vi "Close.vi"(8 "error in (no error)":errorcluster, 11 "Task Base in":refnum<class "Task Base.lvclass">) -> (0 "error out":errorcluster, 3 "Task Base out":refnum<class "Task Base.lvclass">)   [LabVIEW 2023, in "HAL GOOP4.lvlib" / "Task Base.lvclass"]
uses:
  Task Base.lvclass
  Task Base.lvclass/Task Base.ctl
  Measure and Stimulus Subsystems/Measure and Stimulus Subsystems.lvclass
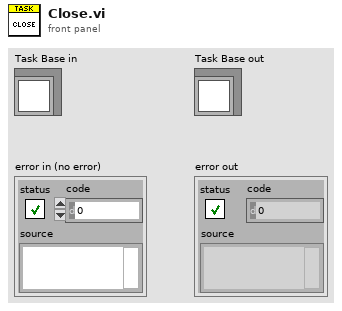
[diagram p1: front panel]
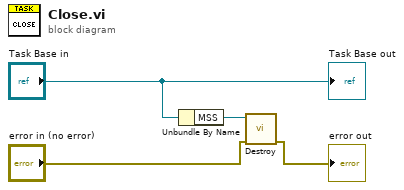
[diagram p0: block diagram]
diagram:
  n1 = Unbundle By Name("Task Base in") -> ("MSS"=w3:refnum<class "Measure and Stimulus Subsystems.lvclass">)
  n2 = call "Destroy.vi"("Error In"="error in (no error)", "reference in"=w3) -> ("Error Out"=→"error out":errorcluster)  [unwired: 8 in, 1 out]
  "Task Base out" <- "Task Base in"
